vi "Ident Req.vi"() -> (3 "String":string)   [LabVIEW 2015]
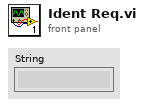
[diagram p1: front panel]
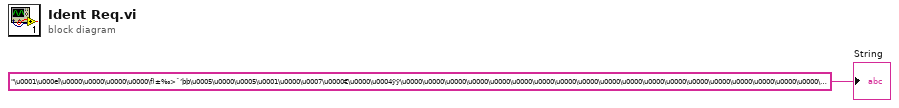
[diagram p0: block diagram]
diagram:
  "String" <- "\u0001\u000eÏ\u0000\u0000\u0000\u0000\f)±‰>ˆ’þþ\u0005\u0000\u0005\u0001\u0000\u0007\u0000€\u0000\u0004ÿÿ\u0000\u0000\u0000\u0000\u0000\u0000\u0000\u0000\u0000\u0000\u0000\u0000\u0000\u0000\u0000\u0000\u0000\u0000\u0000\u0000\u0000\u0000\u0000\u0000\u0000\u0000\u0000\u0000\u0000\u0000\u0000\u0000"
